vi "dcy03.vi"() -> ()   [LabVIEW 2023]
uses:
  parametertype.ctl
  <vilib>/regexp/Match Regular Expression.xnode
  SECoP.lvlib
panel:
  out "log":string
  in  "DLL path":path=path "D:/git-repos/shall-labview/64bit"
  in  "stop":bool
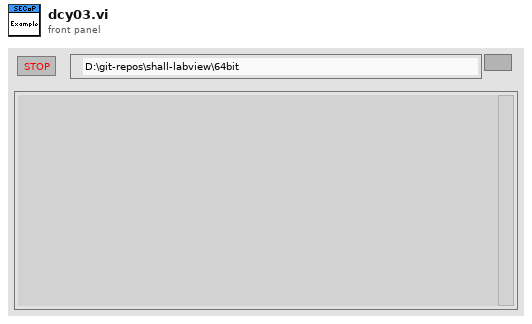
[diagram p1: front panel]
types:
  T1 = typedef "parametertype.ctl" = enum8{"readonly", "readwrite", "command"}
  T2 = cluster{"name":string, "type":T1, "datatype":string, "description":string}[]
  T3 = typedef "SECoP.lvlib/SECoP-libraries.ctl" = cluster{"serverDLL":path, "variantDLL":path, "cleanup_mode":bool, "Context_ID":string}
  T4 = typedef "SECoP.lvlib/SECoP-action.ctl" = enum32{"any action", "read", "change", "do cmd"}
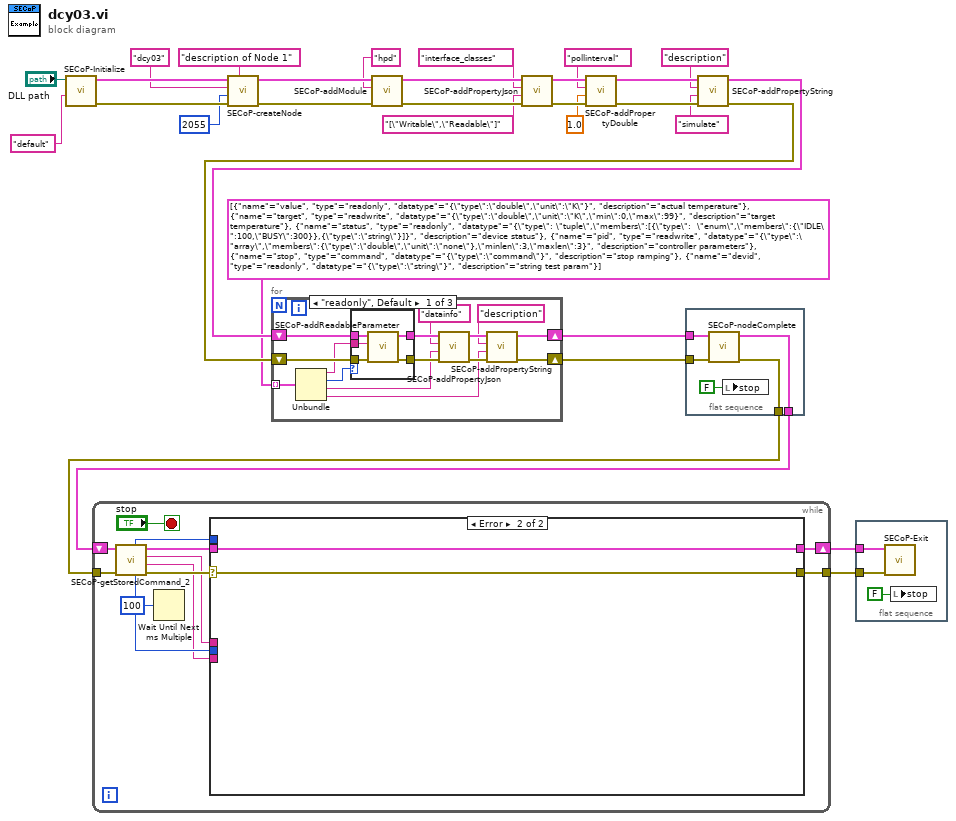
[diagram p0: block diagram]
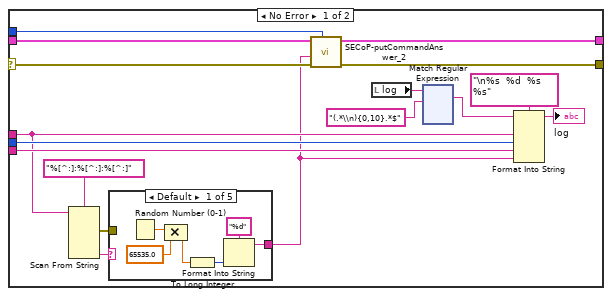
[diagram p2: hidden frame]
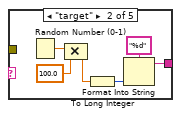
[diagram p3: hidden frame]
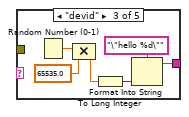
[diagram p4: hidden frame]
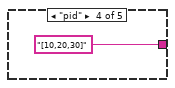
[diagram p5: hidden frame]
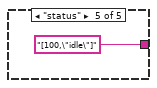
[diagram p6: hidden frame]
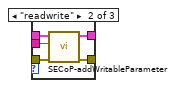
[diagram p7: hidden frame]
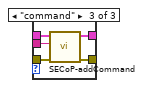
[diagram p8: hidden frame]
diagram:
  n1 = call "SECoP-Initialize.vi"("Context ID (in)"="default", "DLL path (in)"="DLL path") -> ("error out"=w27:errorcluster, "DLL path (out)"=w28:T3)  [unwired: 8 in]
  n2 = while {
    shift-right: [w43] -> w16
    shift-left: w7 -> [w41]
    tunnel: w8 -> [w40]
    tunnel: [w33] -> w15
    stop <- "stop" stop-if-true
    n3 = call "SECoP-getStoredCommand_2.vi"("error in (no error)"=w40, "DLL path (in)"=w41) -> ("error out"=w38:errorcluster, "arguments/setvalue"=w34:string, "command/parameter path"=w35:string, "DLL path (out)"=w39:T3, "action"=w36:T4, "command id"=w37:u64)  [unwired: 4 in]
    n4 = Wait Until Next ms Multiple(millisecond multiple=u32 100) -> ()  [unwired: 1 out]
    n5 = case shown="Error" w38 {
      selector: w38 -> [w60 w198]
      tunnel: w39 -> [w59 w199]
      tunnel: [w58 w199] -> w43
      tunnel: w37 -> [w57 _]
      tunnel: w35 -> [w48 _]
      tunnel: w34 -> [w54 _]
      tunnel: w36 -> [w55 _]
      tunnel: [w56 w198] -> w33
      frame No Error {
        n6 = Scan From String(format string="%[^:]:%[^:]:%[^:]", input string=w48) -> (error out=w45:errorcluster, output 3=w47:string)  [unwired: 7 in, 2 out]
        n7 = case shown="Default" w47 {
          tunnel: [w61 w67 w73 "[10,20,30]" "[100,\"idle\"]"] -> w46
          tunnel: w45 -> [_ _ _ _ _]
          frame Default {
            n8 = Random Number (0-1)() -> (number: 0 to 1=w63:dbl)
            n9 = Compound Arithmetic op=MULTIPLY(w63, 65535.0 ("value")) -> (w65:dbl)
            n10 = To Long Integer(number=w65) -> (32bit integer=w66:i32)
            n11 = Format Into String(format string="%d", w66) -> (resulting string=w61:string)  [unwired: 2 in, 1 out]
          }
          frame "target" {
            n12 = Random Number (0-1)() -> (number: 0 to 1=w69:dbl)
            n13 = Compound Arithmetic op=MULTIPLY(w69, 100.0 ("value")) -> (w71:dbl)
            n14 = To Long Integer(number=w71) -> (32bit integer=w72:i32)
            n15 = Format Into String(format string="%d", w72) -> (resulting string=w67:string)  [unwired: 2 in, 1 out]
          }
          frame "devid" {
            n16 = Random Number (0-1)() -> (number: 0 to 1=w75:dbl)
            n17 = Compound Arithmetic op=MULTIPLY(w75, 65535.0 ("value")) -> (w77:dbl)
            n18 = To Long Integer(number=w77) -> (32bit integer=w78:i32)
            n19 = Format Into String(format string="\"hello %d\"", w78) -> (resulting string=w73:string)  [unwired: 2 in, 1 out]
          }
          frame "pid" {
          }
          frame "status" {
          }
        }
        n20 = call "SECoP-putCommandAnswer_2.vi"("command id"=w57, "error in (no error)"=w60, "value"=w46, "DLL path (in)"=w59) -> ("error out"=w56:errorcluster, "DLL path (out)"=w58:T3)  [unwired: 6 in]
        n21 = local read "log"() -> (w51:string)
        n22 = xnode "Match Regular Expression"("input string"=w51, "regular expression"="(.*\\n){0,10}.*$") -> ("whole match"=w52:string)  [unwired: 4 in, 4 out]
        n23 = Format Into String(format string="\n%s  %d  %s  %s", initial string=w52, w48, w55, w54, w46) -> (resulting string=→"log":string)  [unwired: 1 in, 1 out]
      }
      frame Error {
      }
    }
  }
  n24 = call "SECoP-createNode.vi"("description"="description of Node 1", "error in (no error)"=w27, "TCP port"=u16 2055, "node id"="dcy03" ("id"), "DLL path (in)"=w28) -> ("error out"=w22:errorcluster, "DLL path (out)"=w26:T3)  [unwired: 5 in]
  n25 = call "SECoP-addModule.vi"("error in (no error)"=w22, "module name"="hpd" ("name"), "DLL path (in)"=w26) -> ("error out"=w19:errorcluster, "DLL path (out)"=w20:T3)  [unwired: 7 in]
  n26 = call "SECoP-addPropertyJson.vi"("error in (no error)"=w19, "property value"="[\"Writable\",\"Readable\"]" ("name"), "property name"="interface_classes" ("name"), "DLL path (in)"=w20) -> ("error out"=w11:errorcluster, "DLL path (out)"=w12:T3)  [unwired: 6 in]
  n27 = call "SECoP-addPropertyDouble.vi"("error in (no error)"=w11, "property value"=1.0, "property name"="pollinterval", "DLL path (in)"=w12) -> ("error out"=w31:errorcluster, "DLL path (out)"=w30:T3)  [unwired: 6 in]
  n28 = flat-sequence {
    tunnel: w6 -> [w203]
    tunnel: w5 -> [w202]
    tunnel: [w200] -> w7
    tunnel: [w201] -> w8
    frame #0 {
      n29 = call "SECoP-nodeComplete.vi"("error in (no error)"=w202, "DLL path (in)"=w203) -> ("error out"=w201:errorcluster, "DLL path (out)"=w200:T3)  [unwired: 8 in]
      n30 = local write "stop"(FALSE) -> ()
    }
  }
  n31 = call "SECoP-addPropertyString.vi"("error in (no error)"=w31, "property value"="simulate" ("name"), "property name"="description" ("name"), "DLL path (in)"=w30) -> ("error out"=w3:errorcluster, "DLL path (out)"=w4:T3)  [unwired: 6 in]
  n32 = for {
    tunnel: T2 [{"name"="value", "type"=enum."readonly", "datatype"="{\"type\":\"double\",\"unit\":\"K\"}", "description"="actual temperature"}, {"name"="target", "type"=enum."readwrite", "datatype"="{\"type\":\"double\",\"unit\":\"K\",\"min\":0,\"max\":99}", "description"="target temperature"}, {"name"="status", "type"=enum."readonly", "datatype"="{\"type\": \"tuple\",\"members\":[{\"type\":  \"enum\",\"members\":{\"IDLE\":100,\"BUSY\":300}},{\"type\":\"string\"}]}", "description"="device status"}, {"name"="pid", "type"=enum."readwrite", "datatype"="{\"type\":\"array\",\"members\":{\"type\":\"double\",\"unit\":\"none\"},\"minlen\":3,\"maxlen\":3}", "description"="controller parameters"}, {"name"="stop", "type"=enum."command", "datatype"="{\"type\":\"command\"}", "description"="stop ramping"}, {"name"="devid", "type"=enum."readonly", "datatype"="{\"type\":\"string\"}", "description"="string test param"}] -> [w207] mode=indexing
    shift-right: [w206] -> w6
    shift-left: w4 -> [w216]
    shift-right: [w205] -> w5
    shift-left: w3 -> [w215]
    n33 = Unbundle(w207) -> ("name"=w208:string, "type"=w217:T1, "datatype"=w209:string, "description"=w210:string)
    n34 = case shown="\"readonly\", Default" w217 {
      tunnel: w208 -> [w222 w229 w234]
      tunnel: w216 -> [w224 w228 w233]
      tunnel: [w223 w227 w232] -> w214
      tunnel: [w220 w225 w230] -> w213
      tunnel: w215 -> [w221 w226 w231]
      frame "readonly", Default {
        n35 = call "SECoP-addReadableParameter.vi"("error in (no error)"=w221, "parameter name"=w222, "DLL path (in)"=w224) -> ("error out"=w220:errorcluster, "DLL path (out)"=w223:T3)  [unwired: 7 in]
      }
      frame "readwrite" {
        n36 = call "SECoP-addWritableParameter.vi"("error in (no error)"=w226, "parameter name"=w229, "DLL path (in)"=w228) -> ("error out"=w225:errorcluster, "DLL path (out)"=w227:T3)  [unwired: 7 in]
      }
      frame "command" {
        n37 = call "SECoP-addCommand.vi"("error in (no error)"=w231, "command name"=w234, "DLL path (in)"=w233) -> ("error out"=w230:errorcluster, "DLL path (out)"=w232:T3)  [unwired: 7 in]
      }
    }
    n38 = call "SECoP-addPropertyJson.vi"("error in (no error)"=w213, "property value"=w209, "property name"="datainfo" ("name"), "DLL path (in)"=w214) -> ("error out"=w218:errorcluster, "DLL path (out)"=w219:T3)  [unwired: 6 in]
    n39 = call "SECoP-addPropertyString.vi"("error in (no error)"=w218, "property value"=w210, "property name"="description" ("name"), "DLL path (in)"=w219) -> ("error out"=w205:errorcluster, "DLL path (out)"=w206:T3)  [unwired: 6 in]
  }
  n40 = flat-sequence {
    tunnel: w16 -> [w236]
    tunnel: w15 -> [w235]
    frame #0 {
      n41 = call "SECoP-Exit.vi"("error in (no error)"=w235, "DLL path (in)"=w236) -> ()  [unwired: 9 in, 1 out]
      n42 = local write "stop"(FALSE) -> ()
    }
  }
